vi "IPG Laser Pluse Generator.vi"() -> ()   [LabVIEW 2012]
doc: "Shows how to configure then create an arbitrary waveform."
uses:
  Trap Frequency AFG Control/Public/Agilent 33XXX Series.lvlib
panel:
  out "Offset":dbl
  out "Amplitude":dbl
  in  "Maximum Voltage":dbl=10.0
  in  "Initial Voltage":dbl=2.0
  in  "Final Voltage":dbl=4.0
  out "Frequency":dbl=0.4838
  in  "Trigger Source (0: Internal)":u16(ring)=1 items=["Internal", "External", "Software (bus)"]
  in  "Enable Burst":bool=TRUE
  in  "Burst Mode (0: Triggered)":u16(ring) items=["Triggered", "Gated"]
  out "Simulated WaveForm":dbl[](graph)
  out "Total Time  (<16000)":i32
  in  "Final Keep Time":i32=100
  in  "Fall Down Time":i32=1000
  in  "Rise Up Time":i32=15
  in  "Pulse Width":i32=100
  in  "Inintial Voltage Time":i32=1
  in  "VISA resource name":refnum<visa-resource-name>
  in  "Arbitrary Waveform Name":string="ARB1"
  # "Read me: (Very Important!!!!!!!!!)\n1. This Labview is used to control the IPG laser output power, When you edit this programme make sure the IPG laser is off.\n2. follow the steps, First is the visa address setting; Second is the pulse edit; Third is the output checking; Forth is the trigger set .\n3. The maximum input voltage is 10V, the minmum value is 1V. The total input time must smaller than 16000ms and larger than 8 ms."
  # "IPG Laser Pulse Controller\n                             ----- FORT trap depth control"
  # "Setp 1"
  # "Setp 3"
  # "Setp 2"
  # "(ms)"
  # "Time (ms)"
  # "Voltage (V)"
  # "(Hz)"
  # "(V)"
  # "(V)"
  # "Setp 4"
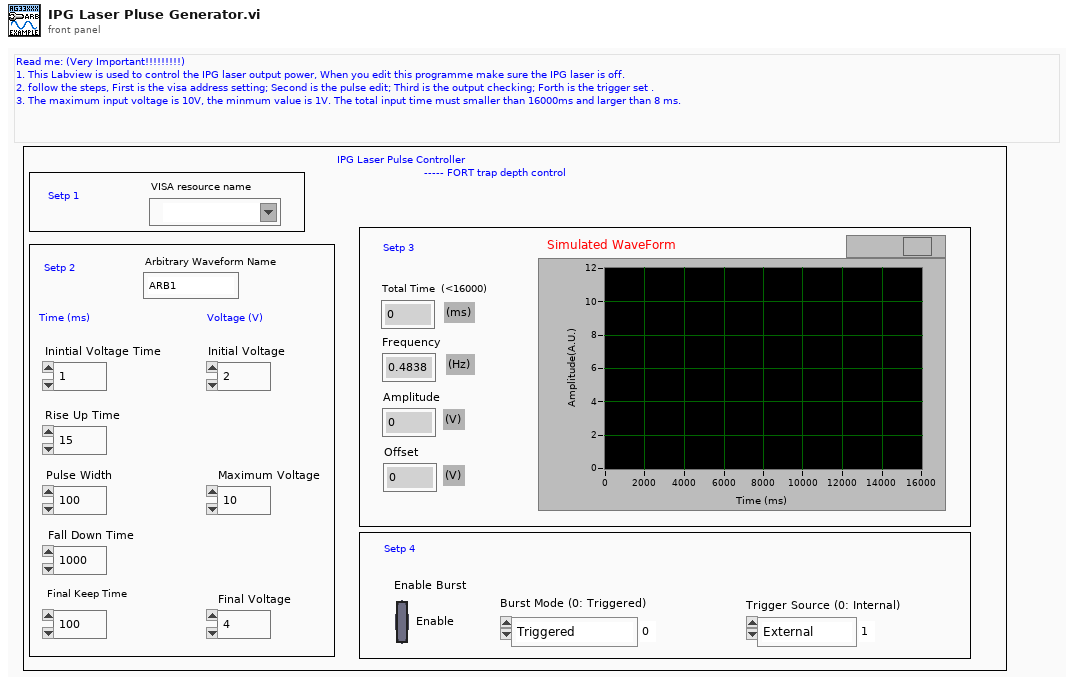
[diagram p1: front panel]
types:
  T1 = cluster{"Baud Rate":u32, "Parity":u16, "Data Bits":u16, "Flow Control":u16}
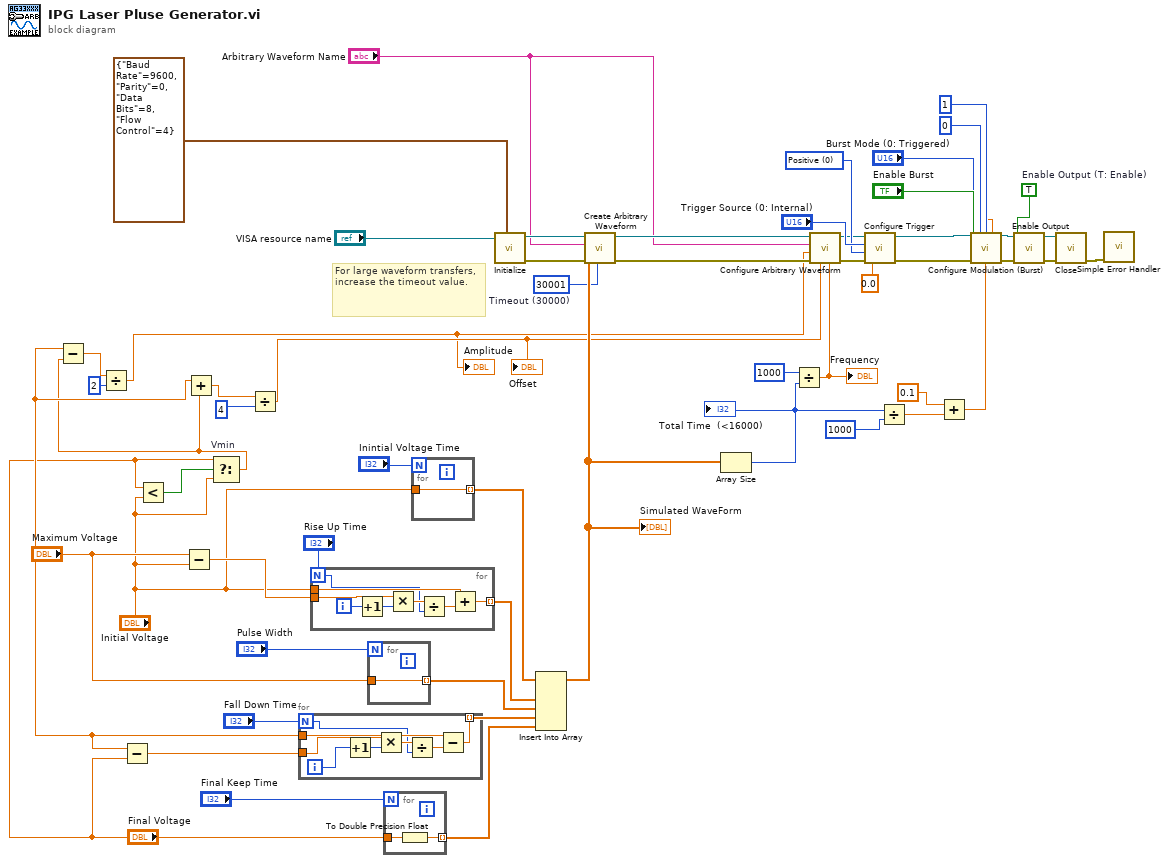
[diagram p0: block diagram]
diagram:
  w40 = u16 0 items=["Positive", "Negative"] ("Slope (0: Positive)")
  w16 = u32 30001  # Timeout (30000)
  w53 = TRUE  # Enable Output (T: Enable)
  # "For large waveform transfers, increase the timeout value."
  n1 = Subtract(x="Maximum Voltage", y="Final Voltage") -> (x-y=w12:dbl)
  n2 = Less?(x="Final Voltage", y="Initial Voltage") -> (x < y?=w11:bool)
  n3 = Subtract(x="Maximum Voltage", y="Initial Voltage") -> (x-y=w14:dbl)
  n4 = Select "Vmin"(t="Final Voltage", s=w11, f="Initial Voltage") -> (s? t:f=w7:dbl)
  n5 = Subtract(x="Maximum Voltage", y=w7) -> (x-y=w10:dbl)
  n6 = Divide(x=w10, y=2) -> (x/y=w1:dbl)
  "Amplitude" <- w1
  n7 = Add(x="Maximum Voltage", y=w7) -> (x+y=w6:dbl)
  n8 = Divide(x=w6, y=4) -> (x/y=w4:dbl)
  "Offset" <- w4
  n9 = for {
    N: "Fall Down Time" -> [w57]
    tunnel: [w62] -> w44 mode=indexing
    tunnel: w12 -> [w59]
    tunnel: "Maximum Voltage" -> [w58]
    i -> [w61]
    n10 = Increment(x=w61) -> (x+1=w60:i32)
    n11 = Multiply(x=w59, y=w60) -> (x*y=w64:dbl)
    n12 = Divide(x=w64, y=w57) -> (x/y=w63:dbl)
    n13 = Subtract(x=w58, y=w63) -> (x-y=w62:dbl)
  }
  n14 = for {
    N: "Rise Up Time" -> [w66]
    tunnel: [w71] -> w48 mode=indexing
    tunnel: "Initial Voltage" -> [w70]
    tunnel: w14 -> [w68]
    i -> [w72]
    n15 = Increment(x=w72) -> (x+1=w69:i32)
    n16 = Multiply(x=w68, y=w69) -> (x*y=w67:dbl)
    n17 = Divide(x=w67, y=w66) -> (x/y=w65:dbl)
    n18 = Add(x=w70, y=w65) -> (x+y=w71:dbl)
  }
  n19 = for {
    N: "Pulse Width" -> [_]
    tunnel: [w73] -> w45 mode=indexing
    tunnel: "Maximum Voltage" -> [w73]
  }
  n20 = for {
    N: "Final Keep Time" -> [_]
    tunnel: [w74] -> w42 mode=indexing
    tunnel: "Final Voltage" -> [w75]
    n21 = To Double Precision Float(number=w75) -> (double precision float=w74:dbl)
  }
  n22 = for {
    N: "Inintial Voltage Time" -> [_]
    tunnel: [w76] -> w46 mode=indexing
    tunnel: "Initial Voltage" -> [w76]
  }
  n23 = call "Initialize.vi"("Serial Configuration"=T1 {"Baud Rate"=9600, "Parity"=0, "Data Bits"=8, "Flow Control"=4}, "VISA resource name"="VISA resource name") -> ("error out"=w18:errorcluster, "VISA resource name out"=w21:refnum<visa-resource-name>)  [unwired: 8 in]
  n24 = Insert Into Array(array=w46, new element #1=w48, new element #2=w45, new element #3=w44, new element #4=w42) -> (w19:dbl[])  [unwired: 1 in]
  "Simulated WaveForm" <- w19
  n25 = call "Create Arbitrary Waveform.vi"("Timeout (10000)"=w16, "error in (no error)"=w18, "Arbitrary Waveform Data"=w19, "Arbitrary Waveform Name (\"ARB1\")"="Arbitrary Waveform Name", "VISA resource name"=w21) -> ("error out"=w17:errorcluster, "VISA resource name out"=w20:refnum<visa-resource-name>)  [unwired: 5 in]
  n26 = Array Size(array=w19) -> (size(s)=w26:i32)
  "Total Time  (<16000)" <- w26
  n27 = Divide(x=1000, y=w26) -> (x/y=w27:dbl)
  "Frequency" <- w27
  n28 = call "Configure Arbitrary Waveform.vi"("Frequency (1000 Hz)"=w27, "Offset (0.00 V)"=w4, "error in (no error)"=w17, "Gain (1.0)"=w1, "Arbitrary Waveform Name (\"ARB1\")"="Arbitrary Waveform Name", "VISA resource name"=w20) -> ("error out"=w38:errorcluster, "VISA resource name out"=w39:refnum<visa-resource-name>)  [unwired: 4 in]
  n29 = call "Configure Trigger.vi"("Delay (0.0 s)"=0.0, "error in (no error)"=w38, "Slope (0: Positive)"=w40, "Trigger Source (0: Internal)"="Trigger Source (0: Internal)", "VISA resource name"=w39) -> ("error out"=w36:errorcluster, "VISA resource name out"=w37:refnum<visa-resource-name>)  [unwired: 5 in]
  n30 = Divide(x=w26, y=1000) -> (x/y=w24:dbl)
  n31 = Add(x=0.1, y=w24) -> (x+y=w22:dbl)
  n32 = call "Configure Modulation (Burst).vi"("VISA resource name"=w37, "Burst Phase (0 deg)"=0, "Burst Count (1)"=1, "Burst Period (1 s)"=w22, "Enable Burst Modulation (T: Enable)"="Enable Burst", "Burst Modulation Mode (0: Triggered)"="Burst Mode (0: Triggered)", "error in (no error)"=w36) -> ("VISA resource name out"=w35:refnum<visa-resource-name>, "error out"=w34:errorcluster)  [unwired: 7 in]
  n33 = call "Enable Output.vi"("error in (no error)"=w34, "Enable Output  (T: Enable)"=w53, "VISA resource name"=w35) -> ("error out"=w55:errorcluster, "VISA resource name out"=w54:refnum<visa-resource-name>)  [unwired: 7 in]
  n34 = call "Close.vi"("error in (no error)"=w55, "VISA resource name"=w54) -> ("error out"=w56:errorcluster)  [unwired: 9 in]
  n35 = call <vilib>:"Simple Error Handler.vi"("error in (no error)"=w56) -> ()  [unwired: 4 in, 5 out]
